vi "SPI Write Bytes Async.vi"(7 "WriteLen":i32, 9 "pWriteData":u8, 10 "SPIIndex":i32, 11 "DevHandle":i32) -> (1 "pWriteData out":u8, 3 "function return":i32)   [LabVIEW 2010, in "usb2spi.lvlib"]
doc: "int WINAPI SPI_WriteBytesAsync(int DevHandle,int SPIIndex,unsigned char *pWriteData,int WriteLen);"
uses:
  usb2spi.lvlib
  USB2XXX.dll
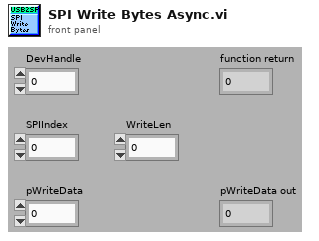
[diagram p1: front panel]
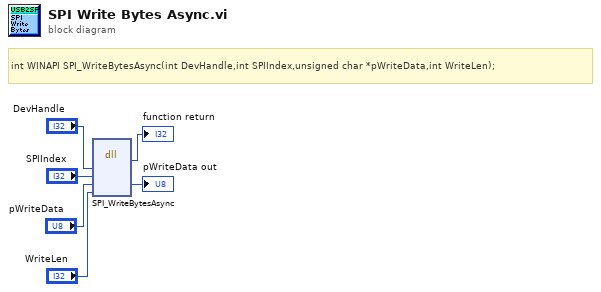
[diagram p0: block diagram]
diagram:
  # "int WINAPI SPI_WriteBytesAsync(int DevHandle,int SPIIndex,unsigned char *pWriteData,int WriteLen);"
  n1 = dll-call lib="G:/OtherWork/USB2XXX_Example/trunk/Labview/PublicFiles/usb2spi/USB2XXX.*" fn="SPI_WriteBytesAsync"("DevHandle"="DevHandle", "SPIIndex"="SPIIndex", "pWriteData"="pWriteData", "WriteLen"="WriteLen") -> (→"function return":i32, "pWriteData"=→"pWriteData out":u8)  [unwired: 6 in, 2 out]
